vi "20220105 main.vi"() -> ()   [LabVIEW 2019]
uses:
  subVI/move/position cluster.ctl
  subVI/move/move array.ctl
  subVI/arduino/Servo/servo option.ctl
panel:
  out "error out":errorcluster
  in  "error in (no error)":errorcluster
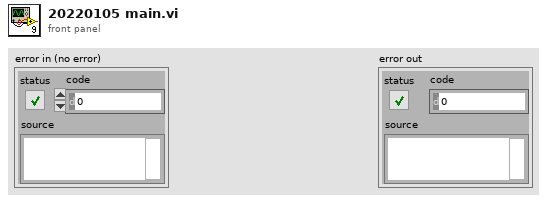
[diagram p1: front panel]
types:
  T1 = typedef "position cluster.ctl" = cluster{"X":dbl, "Y":dbl, "Angle":dbl}
  T2 = enum16{"init", "vision", "vision go to catch", "catch", "A zone to B zone", "B zone put", "goto home"}[]
  T3 = typedef "servo option.ctl" = enum8{"", "put", "catch", "vision-1", "vision-2"}
  T4 = typedef "move array.ctl" = cluster{"X":dbl, "Y":dbl}[]
  T5 = enum16{"init", "vision", "vision go to catch", "catch", "A zone to B zone", "B zone put", "goto home"}
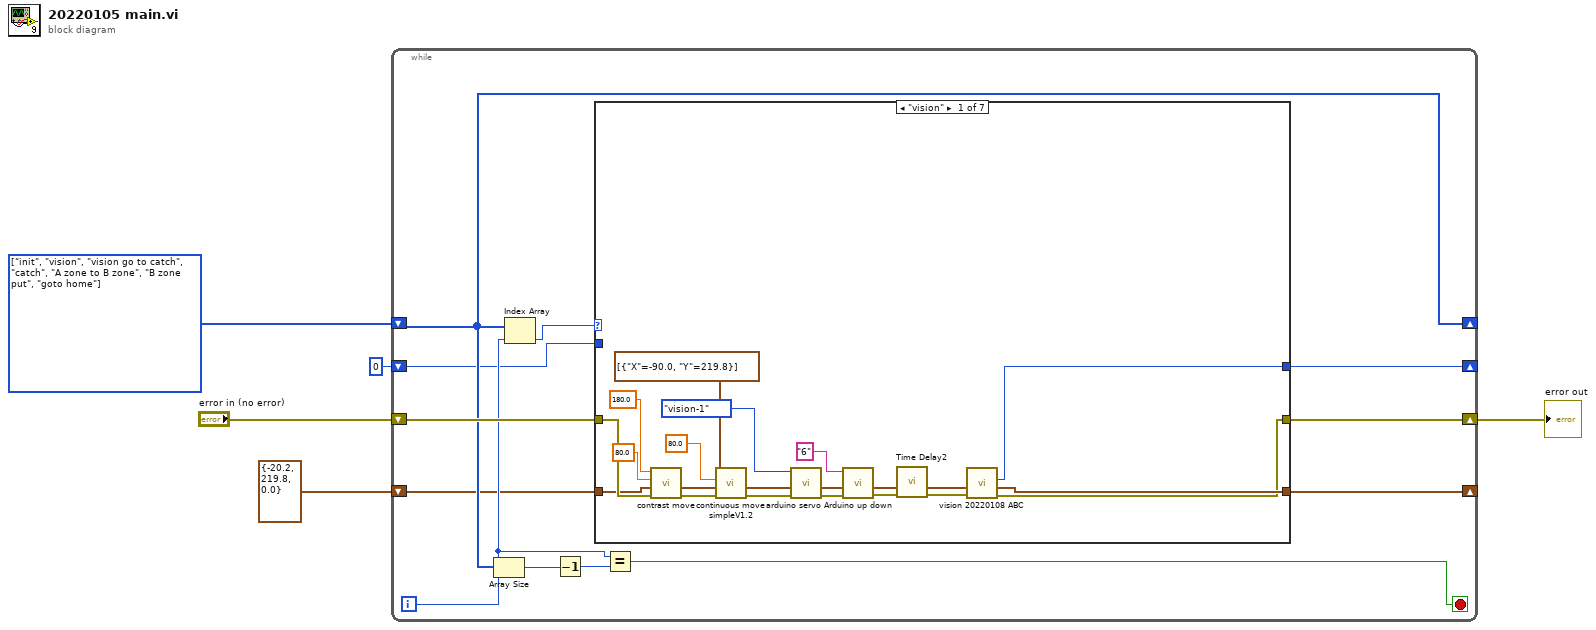
[diagram p0: block diagram]
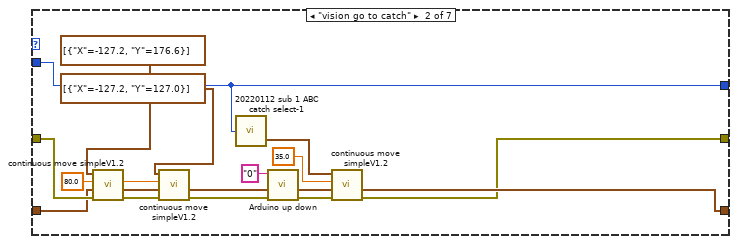
[diagram p2: hidden frame]
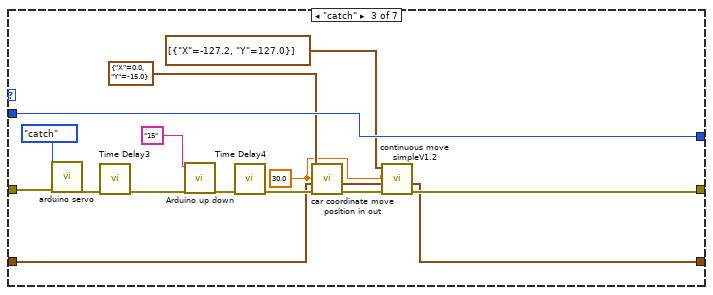
[diagram p3: hidden frame]
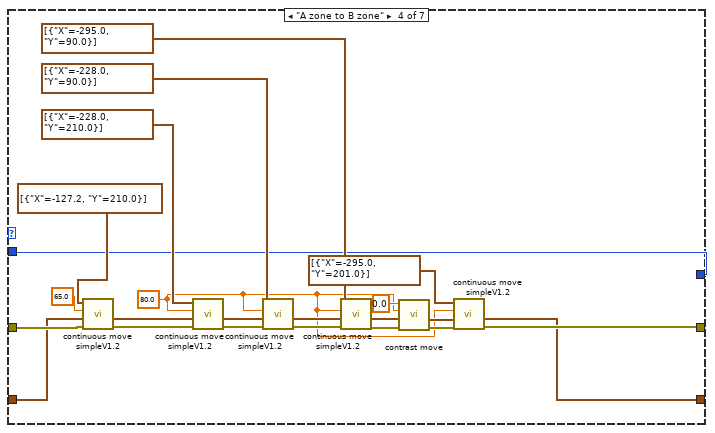
[diagram p4: hidden frame]
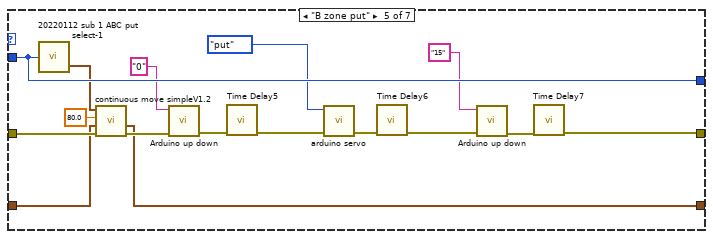
[diagram p5: hidden frame]
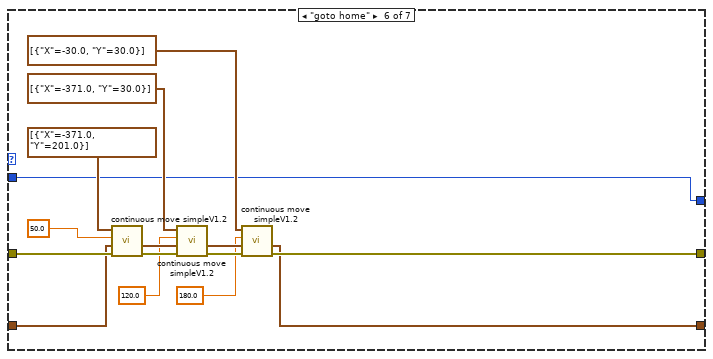
[diagram p6: hidden frame]
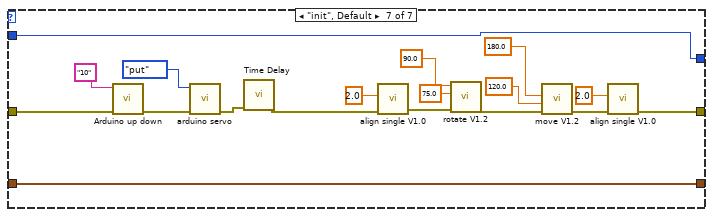
[diagram p7: hidden frame]
diagram:
  w3 = T2 [enum."init", enum."vision", enum."vision go to catch", enum."catch", enum."A zone to B zone", enum."B zone put", enum."goto home"] items=["init", "vision", "vision go to catch", "catch", "A zone to B zone", "B zone put", "goto home"]
  n1 = while {
    shift-right: [w16] -> w4
    shift-left: "error in (no error)" -> [w17]
    shift-right: [w14] -> _
    shift-left: w3 -> [w14]
    shift-right: [w8] -> _
    shift-left: T1 {"X"=-20.2, "Y"=219.8, "Angle"=0.0} ("Position") -> [w9]
    shift-right: [w7] -> _
    shift-left: 0 ("index of wood") -> [w6]
    i -> [w12]
    stop <- w11 stop-if-true
    n2 = Array Size(array=w14) -> (size(s)=w13:i32)
    n3 = Index Array(array=w14, index=w12) -> (element=w15:T5)
    n4 = Decrement(x=w13) -> (x-1=w10:i32)
    n5 = case shown="\"vision\"" w15 {
      tunnel: w17 -> [w34 w50 w66 w89 w104 w120 w124]
      tunnel: [w18 w38 w52 w68 w90 w109 w123] -> w16
      tunnel: w9 -> [w33 w49 w58 w88 w103 w119 w122]
      tunnel: [w26 w39 w51 w67 w92 w108 w122] -> w8
      tunnel: [w19 w43 w60 w76 w105 w107 w121] -> w7
      tunnel: w6 -> [_ w43 w60 w76 w105 w107 w121]
      frame "vision" {
        n6 = call "contrast move.vi"("error in (no error)"=w34, "Position in"=w33, "speed"=80.0, "Target degree"=180.0) -> ("error out"=w30:errorcluster, "Position out"=w29:T1)  [unwired: 6 in]
        n7 = call "continuous move simpleV1.2.vi"("error in (no error)"=w30, "Position"=w29, "Speed"=80.0, "Array"=T4 [{"X"=-90.0, "Y"=219.8}]) -> ("error out"=w25:errorcluster, "Position out"=w26:T1)  [unwired: 6 in]
        n8 = call "arduino servo.vi"("error in (no error)"=w25, "Enum"=servo_option."vision-1") -> ("error out"=w23:errorcluster)  [unwired: 9 in]
        n9 = call "Arduino up down.vi"("error in (no error)"=w23, "Height"="6") -> ("error out"=w21:errorcluster)  [unwired: 9 in]
        n10 = call "Time Delay2"("error in (no error)"=w21) -> ("error out"=w20:errorcluster)  [unwired: 10 in]
        n11 = call "vision 20220108 ABC.vi"("error in"=w20) -> ("error out"=w18:errorcluster, "index of wood"=w19:i32)  [unwired: 5 in]
      }
      frame "vision go to catch" {
        w45 = 80.0 ("Speed")
        n12 = call "continuous move simpleV1.2.vi"("error in (no error)"=w50, "Position"=w49, "Speed"=w45, "Array"=T4 [{"X"=-127.2, "Y"=176.6}]) -> ("error out"=w47:errorcluster, "Position out"=w46:T1)  [unwired: 6 in]
        n13 = call "continuous move simpleV1.2.vi"("error in (no error)"=w47, "Position"=w46, "Speed"=w45, "Array"=T4 [{"X"=-127.2, "Y"=127.0}]) -> ("error out"=w37:errorcluster, "Position out"=w42:T1)  [unwired: 6 in]
        n14 = call "20220112 sub 1 ABC catch select-1.vi"("ABC"=w43) -> ("ABC path out go catch"=w41:cluster{"X":dbl, "Y":dbl}[])  [unwired: 1 in]
        n15 = call "Arduino up down.vi"("error in (no error)"=w37, "Height"="0") -> ("error out"=w36:errorcluster)  [unwired: 9 in]
        n16 = call "continuous move simpleV1.2.vi"("error in (no error)"=w36, "Position"=w42, "Speed"=35.0, "Array"=w41) -> ("error out"=w38:errorcluster, "Position out"=w39:T1)  [unwired: 6 in]
      }
      frame "catch" {
        w53 = 30.0 ("speed")
        n17 = call "arduino servo.vi"("error in (no error)"=w66, "Enum"=servo_option."catch") -> ("error out"=w64:errorcluster)  [unwired: 9 in]
        n18 = call "Time Delay3"("error in (no error)"=w64) -> ("error out"=w63:errorcluster)  [unwired: 10 in]
        n19 = call "Arduino up down.vi"("error in (no error)"=w63, "Height"="15") -> ("error out"=w61:errorcluster)  [unwired: 9 in]
        n20 = call "Time Delay4"("error in (no error)"=w61) -> ("error out"=w59:errorcluster)  [unwired: 10 in]
        n21 = call "car coordinate move position in out.vi"("error in (no error)"=w59, "Position in"=w58, "speed"=w53, "move"=cluster{"X":dbl, "Y":dbl} {"X"=0.0, "Y"=-15.0}) -> ("error out"=w54:errorcluster, "Position out"=w55:T1)  [unwired: 6 in]
        n22 = call "continuous move simpleV1.2.vi"("error in (no error)"=w54, "Position"=w55, "Speed"=w53, "Array"=T4 [{"X"=-127.2, "Y"=127.0}]) -> ("error out"=w52:errorcluster, "Position out"=w51:T1)  [unwired: 6 in]
      }
      frame "A zone to B zone" {
        w69 = 80.0 ("Speed")
        n23 = call "continuous move simpleV1.2.vi"("error in (no error)"=w89, "Position"=w88, "Speed"=65.0, "Array"=T4 [{"X"=-127.2, "Y"=210.0}]) -> ("error out"=w78:errorcluster, "Position out"=w77:T1)  [unwired: 6 in]
        n24 = call "continuous move simpleV1.2.vi"("error in (no error)"=w78, "Position"=w77, "Speed"=w69, "Array"=T4 [{"X"=-228.0, "Y"=210.0}]) -> ("error out"=w82:errorcluster, "Position out"=w83:T1)  [unwired: 6 in]
        n25 = call "continuous move simpleV1.2.vi"("error in (no error)"=w82, "Position"=w83, "Speed"=w69, "Array"=T4 [{"X"=-228.0, "Y"=90.0}]) -> ("error out"=w81:errorcluster, "Position out"=w80:T1)  [unwired: 6 in]
        n26 = call "continuous move simpleV1.2.vi"("error in (no error)"=w81, "Position"=w80, "Speed"=w69, "Array"=T4 [{"X"=-295.0, "Y"=90.0}]) -> ("error out"=w75:errorcluster, "Position out"=w74:T1)  [unwired: 6 in]
        n27 = call "contrast move.vi"("error in (no error)"=w75, "Position in"=w74, "speed"=w69, "Target degree"=0.0) -> ("error out"=w72:errorcluster, "Position out"=w71:T1)  [unwired: 6 in]
        n28 = call "continuous move simpleV1.2.vi"("error in (no error)"=w72, "Position"=w71, "Speed"=w69, "Array"=T4 [{"X"=-295.0, "Y"=201.0}]) -> ("error out"=w68:errorcluster, "Position out"=w67:T1)  [unwired: 6 in]
      }
      frame "B zone put" {
        n29 = call "20220112 sub 1 ABC put select-1.vi"("ABC"=w105) -> ("ABC path out go catch"=w101:cluster{"X":dbl, "Y":dbl}[])  [unwired: 1 in]
        n30 = call "continuous move simpleV1.2.vi"("error in (no error)"=w104, "Position"=w103, "Speed"=80.0, "Array"=w101) -> ("error out"=w100:errorcluster, "Position out"=w92:T1)  [unwired: 6 in]
        n31 = call "Arduino up down.vi"("error in (no error)"=w100, "Height"="0") -> ("error out"=w98:errorcluster)  [unwired: 9 in]
        n32 = call "Time Delay5"("error in (no error)"=w98) -> ("error out"=w97:errorcluster)  [unwired: 10 in]
        n33 = call "arduino servo.vi"("error in (no error)"=w97, "Enum"=servo_option."put") -> ("error out"=w95:errorcluster)  [unwired: 9 in]
        n34 = call "Time Delay6"("error in (no error)"=w95) -> ("error out"=w94:errorcluster)  [unwired: 10 in]
        n35 = call "Arduino up down.vi"("error in (no error)"=w94, "Height"="15") -> ("error out"=w91:errorcluster)  [unwired: 9 in]
        n36 = call "Time Delay7"("error in (no error)"=w91) -> ("error out"=w90:errorcluster)  [unwired: 10 in]
      }
      frame "goto home" {
        n37 = call "continuous move simpleV1.2.vi"("error in (no error)"=w120, "Position"=w119, "Speed"=50.0, "Array"=T4 [{"X"=-371.0, "Y"=201.0}]) -> ("error out"=w116:errorcluster, "Position out"=w115:T1)  [unwired: 6 in]
        n38 = call "continuous move simpleV1.2.vi"("error in (no error)"=w116, "Position"=w115, "Speed"=120.0, "Array"=T4 [{"X"=-371.0, "Y"=30.0}]) -> ("error out"=w113:errorcluster, "Position out"=w112:T1)  [unwired: 6 in]
        n39 = call "continuous move simpleV1.2.vi"("error in (no error)"=w113, "Position"=w112, "Speed"=180.0, "Array"=T4 [{"X"=-30.0, "Y"=30.0}]) -> ("error out"=w109:errorcluster, "Position out"=w108:T1)  [unwired: 6 in]
      }
      frame "init", Default {
        n40 = call "Arduino up down.vi"("error in (no error)"=w124, "Height"="10") -> ("error out"=w128:errorcluster)  [unwired: 9 in]
        n41 = call "arduino servo.vi"("error in (no error)"=w128, "Enum"=enum8{"", "put", "catch"}."put") -> ("error out"=w126:errorcluster)  [unwired: 9 in]
        n42 = call "Time Delay"("error in (no error)"=w126) -> ("error out"=w125:errorcluster)  [unwired: 10 in]
        n43 = call "align single V1.0.vi"("error in (no error)"=w125, "Target (Volt)"=2.0) -> ("error out"=w137:errorcluster)  [unwired: 9 in]
        n44 = call "rotate V1.2.vi"("error in (no error)"=w137, "speed"=75.0, "degree"=90.0) -> ("error out"=w134:errorcluster)  [unwired: 8 in]
        n45 = call "move V1.2.vi"("error in (no error)"=w134, "RPM"=120.0, "Y"=180.0) -> ("error out"=w130:errorcluster)  [unwired: 8 in]
        n46 = call "align single V1.0.vi"("error in (no error)"=w130, "Target (Volt)"=2.0) -> ("error out"=w123:errorcluster)  [unwired: 9 in]
      }
    }
    n47 = Equal?(x=w12, y=w10) -> (x = y?=w11:bool)
  }
  "error out" <- w4
